vi "Test3v6.vi"() -> ()   [LabVIEW 2013]
panel:
  out "String":string
  out "index":i32
  in  "error in":errorcluster
  out "error out":errorcluster
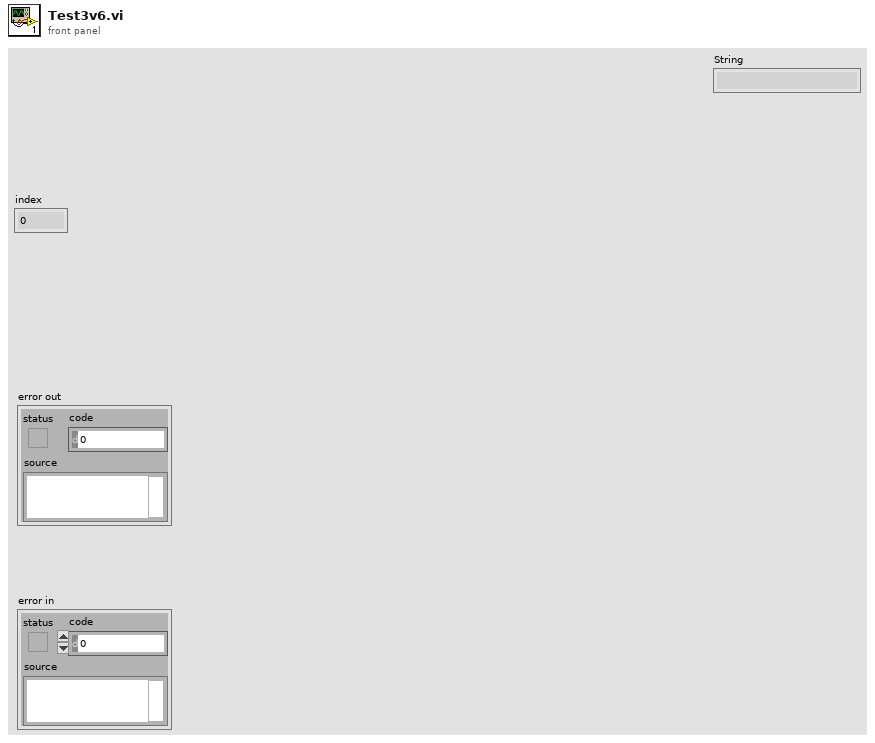
[diagram p1: front panel]
types:
  T1 = enum16{"big-endian, network order", "native, host order", "little-endian"}
  T2 = enum16{"open", "replace", "create", "open or create", "replace or create", "replace or create with confirmation"}
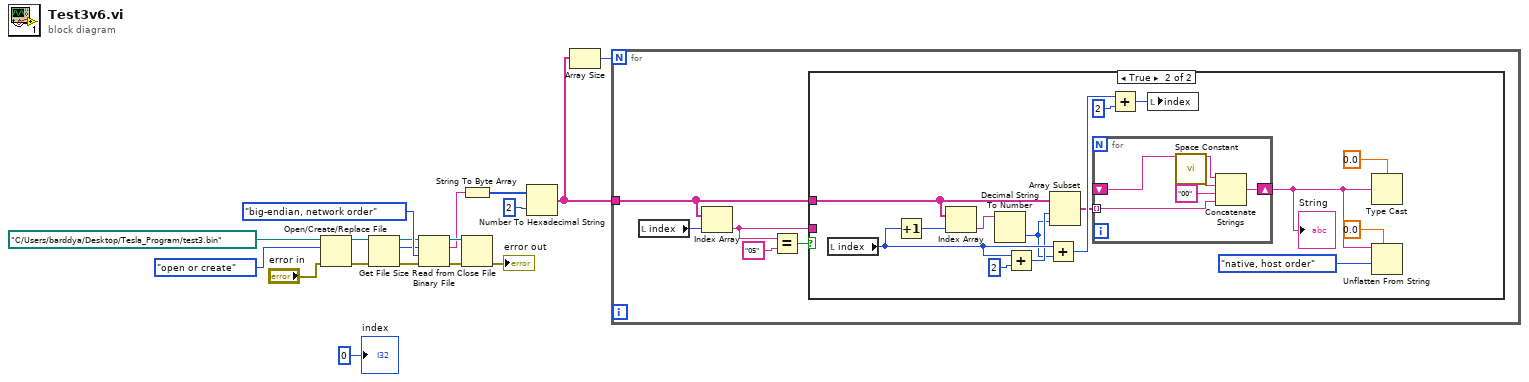
[diagram p0: block diagram]
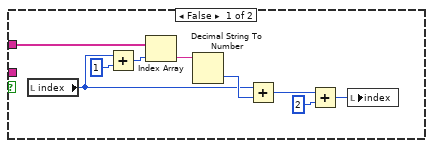
[diagram p2: hidden frame]
diagram:
  n1 = Open/Create/Replace File(file path (use dialog)=path "C:/Users/barddya/Desktop/Tesla_Program/test3.bin", error in="error in", operation (0:open)=T2."open or create") -> (refnum out=w11:refnum<file>, error out=w9:errorcluster)  [unwired: 3 in, 1 out]
  n2 = Get File Size(file=w11, error in=w9) -> (refnum out=w10:refnum<file>, size (in bytes)=w7:i64, 0:w8:errorcluster)
  n3 = Read from Binary File(8:w8, 9:T1."big-endian, network order" ("byte order (0:big-endian, network order)"), 10:w7, 11:w10) -> (0:w14:errorcluster, 2:w6:string, 3:w12:refnum<file>)  [unwired: 2 in, 1 out]
  n4 = String To Byte Array(string=w6) -> (unsigned byte array=w5:u8[])
  n5 = Close File(refnum=w12, error in=w14) -> (error out=→"error out":errorcluster)  [unwired: 1 out]
  n6 = Number To Hexadecimal String(1:2, 2:w5) -> (0:w3:string[])
  n7 = Array Size(array=w3) -> (size(s)=w1:i32)
  n8 = for {
    N: w1 -> [_]
    tunnel: w3 -> [w21]
    n9 = local read "index"() -> (w19:i32)
    n10 = Index Array(array=w21, index=w19) -> (element=w20:string)
    n11 = Equal?(x=w20, y="05") -> (x = y?=w22:bool)
    n12 = case shown="True" w22 {
      tunnel: w21 -> [w30 w44]
      tunnel: w20 -> [_ _]
      frame False {
        n13 = local read "index"() -> (w27:i32)
        n14 = Add(x=w27, y=1) -> (x+y=w28:i32)
        n15 = Index Array(array=w30, index=w28) -> (element=w32:string)
        n16 = Decimal String To Number(string=w32) -> (number=w31:i32)  [unwired: 2 in, 1 out]
        n17 = Add(x=w27, y=w31) -> (x+y=w26:i32)
        n18 = Add(x=w26, y=2) -> (x+y=w24:i32)
        n19 = local write "index"(w24) -> ()
      }
      frame True {
        n20 = local read "index"() -> (w42:i32)
        n21 = Increment(x=w42) -> (x+1=w47:i32)
        n22 = Index Array(array=w44, index=w47) -> (element=w45:string)
        n23 = Decimal String To Number(string=w45) -> (number=w38:i32)  [unwired: 2 in, 1 out]
        n24 = Add(x=w42, y=2) -> (x+y=w40:i32)
        n25 = Add(x=w42, y=w38) -> (x+y=w43:i32)
        n26 = Array Subset(array=w44, index=w40, length=w38) -> (w37:string[])
        n27 = for {
          tunnel: w37 -> [w51] mode=indexing
          shift-right: [w52] -> w33
          shift-left: _ -> [w50]
          n28 = call <vilib>:"Space Constant.vi"() -> ("String"=w48:string)
          n29 = Concatenate Strings(w50, w48, "00", w51) -> (w52:string)
        }
        "String" <- w33
        n30 = Add(x=w43, y=2) -> (x+y=w39:i32)
        n31 = local write "index"(w39) -> ()
        n32 = Type Cast(type=0.0, x=w33) -> ()  [unwired: 1 out]
        n33 = Unflatten From String(type=0.0, binary string=w33, byte order (0:big-endian, network order)=T1."native, host order") -> ()  [unwired: 2 in, 3 out]
      }
    }
  }
  "index" <- 0
